vi "Check Events.vi"(8 "error in (no error)":errorcluster, 11 "RT Data in in":T1 {"Channels"."Voltage"."Ref"."Data Reference" format="%.0x"; "Channels"."Current"."Ref"."Data Reference" format="%.0x"; "Channels"."Read Volt"."Ref" format="%.0x"; "Channels"."Mode"."Ref" format="%.0x"}) -> (0 "error out":errorcluster, 3 "RT Data in out":T1 {"Channels"."Voltage"."Ref"."Data Reference" format="%.0x"; "Channels"."Current"."Ref"."Data Reference" format="%.0x"; "Channels"."Read Volt"."Ref" format="%.0x"; "Channels"."Mode"."Ref" format="%.0x"})   [LabVIEW 2011, in "Switch-DMM Custom Device.lvlib"]
uses:
  Switch-DMM Custom Device.lvlib
  Controls/RT Data.ctl
  Controls/Channels.ctl
  Controls/Single Channel.ctl
  <vilib>/NI Veristand/Custom Device API/Data Reference.ctl
  Controls/Block Channels.ctl
  <vilib>/NI Veristand/Custom Device API/Block Data Reference.ctl
  Controls/Communication.ctl
  Controls/Async Status.ctl
  Controls/Async State.ctl
  Controls/Async Command.ctl
  Controls/Async Events.ctl
  <vilib>/NI Veristand/Custom Device API/Global Data Refs.vi
  <vilib>/NI Veristand/Custom Device API/Custom Device API.lvlib
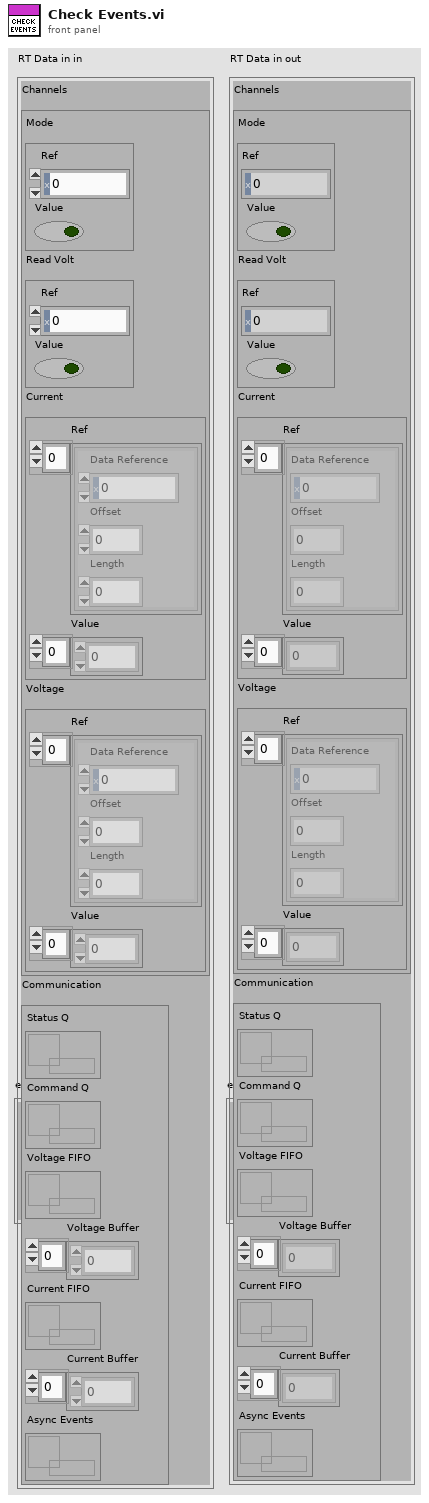
[diagram p1: front panel]
types:
  T1 = typedef "Switch-DMM Custom Device.lvlib/RT Data.ctl" = cluster{"Channels":T2, "Communication":T7}
  T2 = typedef "Switch-DMM Custom Device.lvlib/Channels.ctl" = cluster{"Mode":T3, "Read Volt":T3, "Current":T5, "Voltage":T5}
  T3 = typedef "Switch-DMM Custom Device.lvlib/Single Channel.ctl" = cluster{"Ref":T4, "Value":bool}
  T4 = typedef "Custom Device API.lvlib/Data Reference.ctl" = i32
  T5 = typedef "Switch-DMM Custom Device.lvlib/Block Channels.ctl" = cluster{"Ref":T6[], "Value":dbl[]}
  T6 = typedef "Custom Device API.lvlib/Block Data Reference.ctl" = cluster{"Data Reference":T4, "Offset":i32, "Length":i32}
  T7 = typedef "Switch-DMM Custom Device.lvlib/Communication.ctl" = cluster{"Status Q":refnum<queue>, "Command Q":refnum<queue>, "Voltage FIFO":refnum<k33>, "Voltage Buffer":dbl[], "Current FIFO":refnum<k33>, "Current Buffer":dbl[], "Async Events":refnum<queue>}
  T8 = typedef "Switch-DMM Custom Device.lvlib/Async Events.ctl" = enum16{"None", "Over Current", "Volt Read Done"}
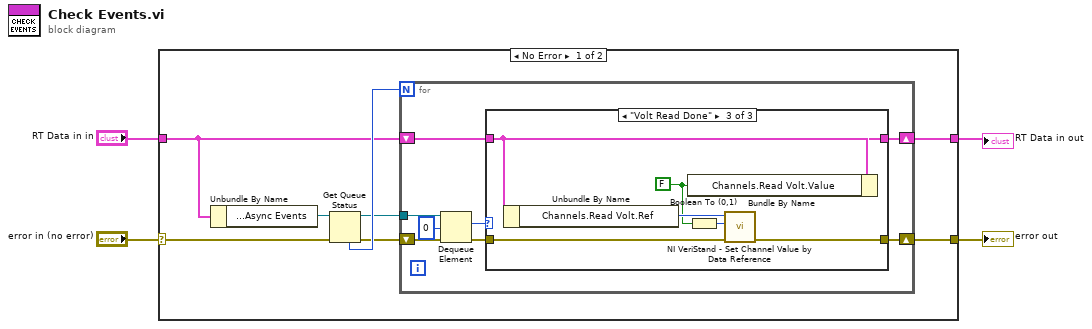
[diagram p0: block diagram]
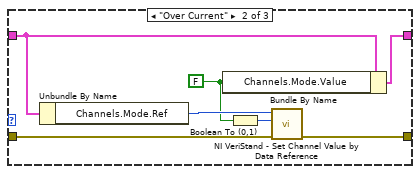
[diagram p3: hidden frame]
diagram:
  n1 = case shown="No Error" "error in (no error)" {
    selector: "error in (no error)" -> [w12 w37]
    tunnel: "RT Data in in" -> [w7 w38]
    tunnel: [w6 w38] -> w3
    tunnel: [w5 w37] -> w4
    frame No Error {
      n2 = Unbundle By Name(w7) -> ("Communication.Async Events"=w11:refnum<queue>)
      n3 = Get Queue Status(queue=w11, error in (no error)=w12) -> (queue out=w8:refnum<queue>, error out=w9:errorcluster, # elements in queue=w10:i32)  [unwired: 1 in, 5 out]
      n4 = for {
        N: w10 -> [_]
        shift-right: [w13] -> w5
        shift-left: w9 -> [w18]
        tunnel: w8 -> [w20]
        shift-right: [w14] -> w6
        shift-left: w7 -> [w15]
        n5 = Dequeue Element(queue=w20, timeout in ms (-1)=0, error in (no error)=w18) -> (element=w17:T8, error out=w16:errorcluster)  [unwired: 2 out]
        n6 = case shown="\"Volt Read Done\"" w17 {
          tunnel: w16 -> [w21 w27 w34]
          tunnel: w15 -> [w22 w28 w35]
          tunnel: [w22 w26 w33] -> w14
          tunnel: [w21 w25 w32] -> w13
          frame "None", Default {
          }
          frame "Over Current" {
            w23 = FALSE
            n7 = Unbundle By Name(w28) -> ("Channels.Mode.Ref"=w29:T4)
            n8 = Bundle By Name(cluster=w28, "Channels.Mode.Value"=w23) -> (w26:T1)
            n9 = Boolean To (0,1)(Boolean=w23) -> (0, 1=w24:i16)
            n10 = call <vilib>:"NI VeriStand - Set Channel Value by Data Reference.vi"("error in (no error)"=w27, "Value"=w24, "Data Reference in"=w29) -> ("error out"=w25:errorcluster)  [unwired: 8 in]
          }
          frame "Volt Read Done" {
            w31 = FALSE
            n11 = Unbundle By Name(w35) -> ("Channels.Read Volt.Ref"=w36:T4)
            n12 = Bundle By Name(cluster=w35, "Channels.Read Volt.Value"=w31) -> (w33:T1)
            n13 = Boolean To (0,1)(Boolean=w31) -> (0, 1=w30:i16)
            n14 = call <vilib>:"NI VeriStand - Set Channel Value by Data Reference.vi"("error in (no error)"=w34, "Value"=w30, "Data Reference in"=w36) -> ("error out"=w32:errorcluster)  [unwired: 8 in]
          }
        }
      }
    }
    frame Error {
    }
  }
  "error out" <- w4
  "RT Data in out" <- w3
